vi "Load Plugin.vi"(6 "timeout (ms)":i32=5000, 8 "error in":errorcluster, 9 "Plugin Path":string, 10 "Plugin Name":string, 11 "gRPC ID in":T1) -> (0 "error out":errorcluster, 3 "gRPC ID out":T1)   [LabVIEW 2021, in "CIFPluginLoaderClientWrapper.lvlib"]
uses:
  CIFPluginLoaderClientWrapper.lvlib
  CIF_PluginLoader_client/CIF_PluginLoader_client.lvlib
  CIF_PluginLoader_client/RPC Messages/cif_pluginloader_LoadConfig.ctl
  CIF_PluginLoader_client/RPC Messages/cif_manager_PluginName.ctl
  <vilib>/gRPC/LabVIEW gRPC Library/Shared/grpcId.ctl
  <vilib>/gRPC/LabVIEW gRPC Library/grpc-lvsupport-release.lvlib
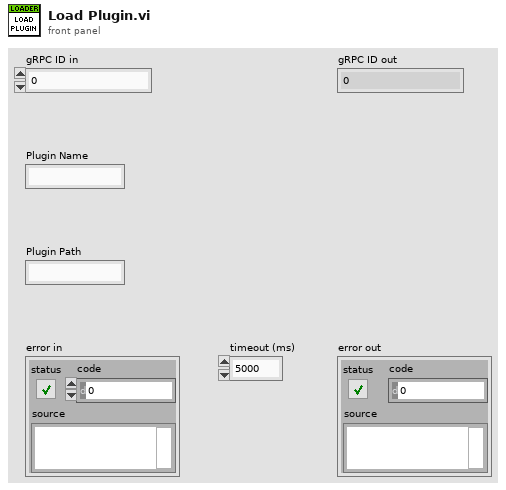
[diagram p1: front panel]
types:
  T1 = typedef "grpc-lvsupport-release.lvlib/grpcId.ctl" = u64
  T2 = typedef "CIF_PluginLoader_client.lvlib/cif_pluginloader_LoadConfig.ctl" = cluster{"plugin_name":T3, "path":string}
  T3 = typedef "CIF_PluginLoader_client.lvlib/cif_manager_PluginName.ctl" = cluster{"plugin_name":string}
  T4 = typedef "CIF_PluginLoader_client.lvlib/cif_common_Status.ctl" = cluster{"code":i32, "message":string}
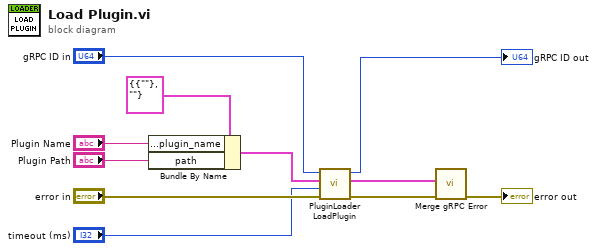
[diagram p0: block diagram]
diagram:
  n1 = Bundle By Name(cluster=T2 {"plugin_name"={"plugin_name"=""}, "path"=""} ("Request Data"), "plugin_name.plugin_name"="Plugin Name", "path"="Plugin Path") -> (w1:T2)
  n2 = call "PluginLoader LoadPlugin.vi"("error in"="error in", "timeout (ms)"="timeout (ms)", "Request Data"=w1, "gRPC ID"="gRPC ID in") -> ("error out"=w7:errorcluster, "Response Data"=w5:T4, "gRPC ID out"=→"gRPC ID out":T1)  [unwired: 5 in]
  n3 = call "Merge gRPC Error.vi"("error in (no error)"=w7, "gRPC Error"=w5) -> ("error out"=→"error out":errorcluster)  [unwired: 9 in]
